vi "Rate Locker.vi"(3 "LockToLS":T1, 4 "LSCfg.Rate":dbl, 5 "HSCfg.Rate":dbl) -> (0 "LSCfg.ReadBlk":i32, 1 "LSCfg.Rate":dbl, 2 "HS Block Size":i32)   [LabVIEW 2012, in "Configuration Grandmaster.lvlib" / "ChassisCfg.lvclass"]
uses:
  ChassisCfg.lvclass
  Common/Controls/LS Lock Sizes.ctl
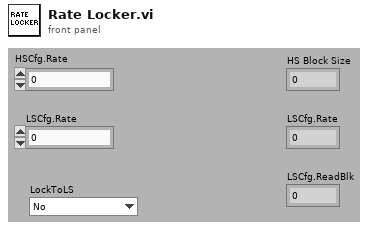
[diagram p1: front panel]
types:
  T1 = typedef "LS Lock Sizes.ctl" = enum16{"No", "250ms", "500ms", "1s"}
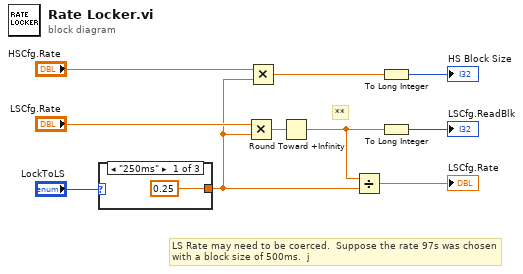
[diagram p0: block diagram]
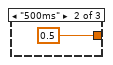
[diagram p2: hidden frame]
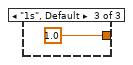
[diagram p3: hidden frame]
diagram:
  # "**"
  # "LS Rate may need to be coerced.  Suppose the rate 97s was chosen\nwith a block size of 500ms.  j"
  n1 = case shown="\"250ms\"" "LockToLS" {
    tunnel: [0.25 0.5 1.0] -> w2
    frame "250ms" {
    }
    frame "500ms" {
    }
    frame "1s", Default {
    }
  }
  n2 = Multiply(x="LSCfg.Rate", y=w2) -> (x*y=w6:dbl)
  n3 = Multiply(x="HSCfg.Rate", y=w2) -> (x*y=w5:dbl)
  n4 = Round Toward +Infinity(x=w6) -> (ceil(x): smallest int >= x=w8:dbl)
  n5 = Divide(x=w8, y=w2) -> (x/y=→"LSCfg.Rate":dbl)
  n6 = To Long Integer(number=w5) -> (32bit integer=→"HS Block Size":i32)
  n7 = To Long Integer(number=w8) -> (32bit integer=→"LSCfg.ReadBlk":i32)
